vi "Teleop.vi"(10 "Match Info":T1={"Autonomous Elapsed Seconds"=0.0, "TeleOp Elapsed Seconds"=0.0, "Disabled Elapsed Seconds"=0.0, "Visited Autonomous"=FALSE, "Visited TeleOp"=FALSE, "Visited Disabled"=FALSE, "Autonomous Settings"={"Autonomous Style"=enum."Independent", "VI Refnum"=refnum}}, 11 "Call Context":T2) -> ()   [LabVIEW 2016]
doc: "This VI is called for each TeleOp packet received from the DS where the robot is not disabled. It is often used to read from the joysticks and update I/O or to update setpoints for timed control loops. It should complete and return within 20 milliseconds or it may miss DS packets."
uses:
  <vilib>/Rock Robotics/WPI/DriverStation/WPI_DriverStationDerivedRobotMode.ctl
  <vilib>/Rock Robotics/WPI/DriverStation/WPI_DriverStationMatch Info.ctl
  <vilib>/Rock Robotics/WPI/Solenoid/WPI_SolenoidValue.ctl
  <vilib>/Rock Robotics/WPI/Utilities/WPI_GetSetVariantRefNum.vi
  <vilib>/Rock Robotics/Network Tables/NT Write Boolean Array.vi
  <vilib>/Rock Robotics/Network Tables/NT Write Numeric Array.vi
  <vilib>/Rock Robotics/Network Tables/NT Read Boolean.vi
  <vilib>/Rock Robotics/Network Tables/NT Read Number.vi
  <vilib>/Rock Robotics/WPI/Solenoid/WPI_SolenoidSetEnum.vi
  <vilib>/Rock Robotics/Network Tables/NT Write Boolean.vi
  Robot Global Data.vi
  <vilib>/Rock Robotics/WPI/RobotDrive/WPI_RobotDriveArcadeDrive_Standard(NoSaturation).vi
panel:
  out "Sample Slider 0":dbl(slide) scale=0.0..5.0
  out "Sample Boolean 1":bool
  out "Sample Boolean 0":bool
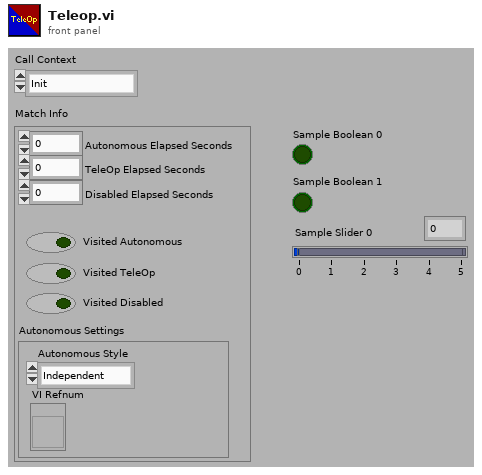
[diagram p1: front panel]
types:
  T1 = typedef "WPI_DriverStationMatch Info.ctl" = cluster{"Autonomous Elapsed Seconds":dbl, "TeleOp Elapsed Seconds":dbl, "Disabled Elapsed Seconds":dbl, "Visited Autonomous":bool, "Visited TeleOp":bool, "Visited Disabled":bool, "Autonomous Settings":cluster{"Autonomous Style":enum16{"Iterative", "Independent"}, "VI Refnum":refnum<vi>}}
  T2 = typedef "WPI_DriverStationDerivedRobotMode.ctl" = enum16{"Init", "Execute", "Stop"}
  T3 = typedef "WPI_SolenoidValue.ctl" = enum16{"Off", "On", "Forward", "Reverse"}
  T4 = typedef "WPI_MotorControlDeviceRef.ctl" = cluster{"DeviceStatus":errorcluster, "Type":T5, "PWM":cluster{"PWM Channel":T6, "DeadBand":T7}, "CAN":cluster{"Device Number":u8, "SetOutput VI Ref":variant, "GetOutput VI Ref":variant, "Enable VI Ref":variant, "Disable VI Ref":variant, "Data":variant}, "Invert":bool}
  T5 = typedef "WPI_MotorControlType.ctl" = enum16{"PWM", "CAN"}
  T6 = typedef "FPGA_DIOPWMChannel.ctl" = enum8{"PWM 0", "PWM 1", "PWM 2", "PWM 3", "PWM 4", "PWM 5", "PWM 6", "PWM 7", "PWM 8", "PWM 9", "PWM MXP 0", "PWM MXP 1", "PWM MXP 2", "PWM MXP 3", "PWM MXP 4", "PWM MXP 5", "PWM MXP 6", "PWM MXP 7", "PWM MXP 8", "PWM MXP 9", "Invalid"}
  T7 = typedef "WPI_PWMDeadband.ctl" = cluster{"Name":string, "maxPositivePwm":i32, "minPositivePwm":i32, "centerPwm":i32, "maxNegativePwm":i32, "minNegativePwm":i32, "angularRange":u16}
  T8 = typedef "WPI_JoystickDevRef.ctl" = cluster{"Device":T9}
  T9 = typedef "WPI_JoystickDeviceEnum.ctl" = enum16{"USB 0", "USB 1", "USB 2", "USB 3", "USB 4", "USB 5"}
  T10 = typedef "WPI_RobotDriveDevRef.ctl" = cluster{"DevStatus":errorcluster, "Motors[]":T4[], "Square Inputs":bool, "Max Output":dbl}
  T11 = typedef "WPI_SolenoidDevRef.ctl" = cluster{"DevStatus":errorcluster, "Pneumatics Control Module":u8, "Forward Solenoid Channel":T12, "Reverse Solenoid Channel":T12}
  T12 = typedef "WPI_SolenoidChannel.ctl" = enum8{"Solenoid 0", "Solenoid 1", "Solenoid 2", "Solenoid 3", "Solenoid 4", "Solenoid 5", "Solenoid 6", "Solenoid 7", "Invalid"}
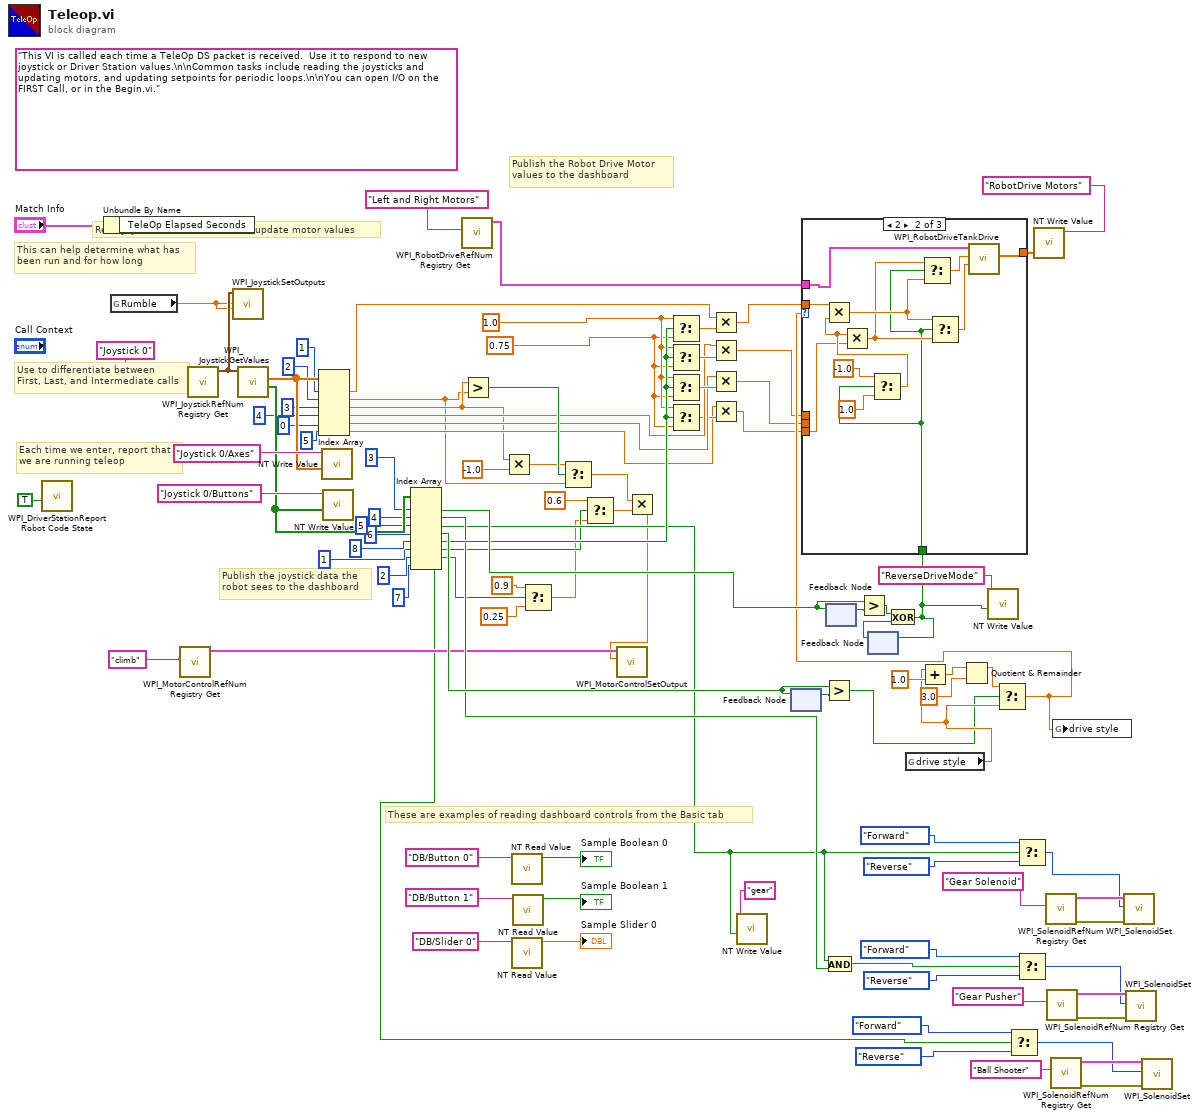
[diagram p0: block diagram]
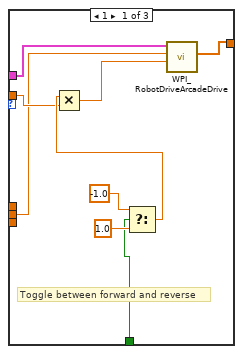
[diagram p2: hidden frame]
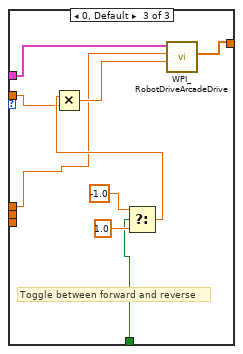
[diagram p3: hidden frame]
diagram:
  w40 = 0.75 ("f")
  w41 = 1.0 ("t")
  (unwired) "This VI is called each time a TeleOp DS packet is received.  Use it to respond to new joystick or Driver Station values.\n\nCommon tasks include reading the joysticks and updating motors, and updating setpoints for periodic loops.\n\nYou can open I/O on the FIRST Call, or in the Begin.vi."
  # "Publish the Robot Drive Motor\nvalues to the dashboard"
  # "These are examples of reading dashboard controls from the Basic tab"
  # "Publish the joystick data the\nrobot sees to the dashboard"
  # "Each time we enter, report that\nwe are running teleop"
  # "Use to differentiate between\nFirst, Last, and Intermediate calls"
  # "This can help determine what has\nbeen run and for how long"
  # "Read Joystick X and Y values and update motor values"
  n1 = call <vilib>:"WPI_DriverStationReport Robot Code State.vi"("TeleOp"=TRUE ("Autonomous")) -> ()  [unwired: 10 in, 1 out]
  n2 = Unbundle By Name("Match Info") -> ()  [unwired: 1 out]
  n3 = global read "Robot Global Data.vi" "Rumble"() -> (w22:dbl)
  n4 = call <vilib>:"WPI_MotorControlRefNum Registry Get.vi"("refnum name"="climb") -> ("MotorControlDevRef"=w16:T4)  [unwired: 9 in, 1 out]
  n5 = call <vilib>:"WPI_JoystickRefNum Registry Get.vi"("refnum name"="Joystick 0") -> ("JoystickDevRef"=w23:T8)  [unwired: 1 in, 9 out]
  n6 = call <vilib>:"WPI_JoystickSetOutputs.vi"("Right Rumble"=w22, "Left Rumble"=w22, "JoystickDevRef"=w23) -> ()  [unwired: 7 in, 2 out]
  n7 = call <vilib>:"WPI_JoystickGetValues.vi"("JoystickDevRef"=w23) -> ("Buttons"=w80:bool[], "Axes"=w96:dbl[])  [unwired: 6 in, 3 out]
  n8 = Index Array(array=w96, index #1=1 ("index"), index #2=2 ("index"), index #3=3 ("index"), index #4=4 ("index"), index #5=0 ("index"), index #6=5 ("index")) -> (element #1=w44:dbl, element #2=w24:dbl, element #3=w25:dbl, element #4=w39:dbl, element #5=w38:dbl, element #6=w36:dbl)
  n9 = call-poly <vilib>:"NT Write Value.vi"("Numeric Array"=w96, "Name"="Joystick 0/Axes") -> ()  [unwired: 9 in, 1 out]
  n10 = call-poly <vilib>:"NT Write Value.vi"("Boolean Array"=w80, "Name"="Joystick 0/Buttons") -> ()  [unwired: 9 in, 1 out]
  n11 = Index Array(array=w80, index #1=3 ("index"), index #2=4 ("index"), index #3=5 ("index"), index #4=6 ("index"), index #5=8 ("index"), index #6=1 ("index"), index #7=2 ("index"), index #8=7 ("index")) -> (element #1=w59:bool, element #2=w28:bool, element #3=w27:bool, element #4=w58:bool, element #5=w45:bool, element #6=w18:bool, element #7=w12:bool, element #8=w1:bool)
  n12 = call <vilib>:"WPI_RobotDriveRefNum Registry Get.vi"("refnum name"="Left and Right Motors") -> ("RobotDriveDevRef"=w75:T10)  [unwired: 1 in, 9 out]
  n13 = Greater?(x=w25, y=w24) -> (0:w62:bool)
  n14 = Multiply(x=w25, y=-1.0) -> (x*y=w26:dbl)
  n15 = call-poly <vilib>:"NT Read Value.vi"("Name"="DB/Button 0" ("refnum name")) -> ("Boolean"=→"Sample Boolean 0":bool)  [unwired: 9 in, 1 out]
  n16 = call-poly <vilib>:"NT Read Value.vi"("Name"="DB/Slider 0" ("refnum name")) -> ("Numeric"=→"Sample Slider 0":dbl)  [unwired: 9 in, 1 out]
  n17 = call-poly <vilib>:"NT Read Value.vi"("Name"="DB/Button 1" ("refnum name")) -> ("Boolean"=→"Sample Boolean 1":bool)  [unwired: 9 in, 1 out]
  n18 = Select(t=0.9, s=w12, f=0.25) -> (s? t:f=w9:dbl)
  n19 = Select(t=w26, s=w62, f=w24) -> (s? t:f=w20:dbl)
  n20 = Select(t=0.6, s=w18, f=w9) -> (s? t:f=w21:dbl)
  n21 = Multiply(x=w20, y=w21) -> (x*y=w13:dbl)
  n22 = call <vilib>:"WPI_MotorControlSetOutput.vi"("Output"=w13, "MotorControlDevRef"=w16) -> ()  [unwired: 7 in, 3 out]
  n23 = Select(t=w41, s=w45, f=w40) -> (s? t:f=w47:dbl)
  n24 = Select(t=w41, s=w45, f=w40) -> (s? t:f=w43:dbl)
  n25 = Select(t=w41, s=w45, f=w40) -> (s? t:f=w42:dbl)
  n26 = Select(t=w41, s=w45, f=w40) -> (s? t:f=w37:dbl)
  n27 = Multiply(x=w44, y=w47) -> (x*y=w46:dbl)
  n28 = Multiply(x=w39, y=w43) -> (x*y=w35:dbl)
  n29 = Multiply(x=w38, y=w42) -> (x*y=w34:dbl)
  n30 = Multiply(x=w36, y=w37) -> (x*y=w33:dbl)
  n31 = call-poly <vilib>:"NT Write Value.vi"("Boolean"=w27, "Name"="gear") -> ()  [unwired: 9 in, 1 out]
  n32 = feedback #1() -> (w60:bool)  [unwired: 1 in]
  n33 = feedback-in #1(w58) -> ()
  n34 = Greater?(x=w58, y=w60) -> (0:w50:bool)
  n35 = And(x=w27, y=w28) -> (x .and. y?=w29:bool)
  n36 = feedback #2() -> (w69:bool)  [unwired: 1 in]
  n37 = feedback-in #2(w59) -> ()
  n38 = Greater?(x=w59, y=w69) -> (0:w68:bool)
  n39 = feedback #3() -> (w70:bool)  [unwired: 1 in]
  n40 = Exclusive Or(1:w70, 2:w68) -> (0:w67:bool)
  n41 = feedback-in #3(w67) -> ()
  n42 = global read "Robot Global Data.vi" "drive style"() -> (w56:dbl)
  n43 = Add(x=w56, y=1.0) -> (x+y=w53:dbl)
  n44 = Quotient & Remainder(x=w53, y=3.0) -> (x-y*floor(x/y)=w55:dbl)  [unwired: 1 out]
  n45 = call-poly <vilib>:"NT Write Value.vi"("Boolean"=w67, "Name"="ReverseDriveMode") -> ()  [unwired: 9 in, 1 out]
  n46 = Select(t=w55, s=w50, f=w56) -> (s? t:f=w52:dbl)
  n47 = case shown="2" w52 {
    tunnel: w75 -> [w110 w115 w131]
    tunnel: w46 -> [w104 w114 w124]
    tunnel: [w111 w112 w132] -> w73
    tunnel: w35 -> [_ _ w125]
    tunnel: w67 -> [w105 w116 w126]
    tunnel: w34 -> [w103 _ _]
    tunnel: w33 -> [_ w113 _]
    frame 1 {
      # "Toggle between forward and reverse"
      n48 = Select(t=-1.0, s=w105, f=1.0) -> (s? t:f=w107:dbl)
      n49 = Multiply(x=w107, y=w104) -> (x*y=w106:dbl)
      n50 = call-poly <vilib>:"WPI_RobotDriveArcadeDrive.vi"("Y axis value"=w106, "X axis value"=w103, "RobotDriveDevRef"=w110) -> ("Motor Values"=w111:dbl[])  [unwired: 6 in, 2 out]
    }
    frame 2 {
      n51 = Select(t=-1.0, s=w116, f=1.0) -> (s? t:f=w117:dbl)
      n52 = Multiply(x=w114, y=w117) -> (x*y=w120:dbl)
      n53 = Multiply(x=w117, y=w113) -> (x*y=w118:dbl)
      n54 = Select(t=w118, s=w116, f=w120) -> (s? t:f=w119:dbl)
      n55 = Select(t=w120, s=w116, f=w118) -> (s? t:f=w121:dbl)
      n56 = call <vilib>:"WPI_RobotDriveTankDrive.vi"("Right axis value"=w121, "Left axis value"=w119, "RobotDriveDevRef"=w115) -> ("Motor Values"=w112:dbl[])  [unwired: 6 in, 2 out]
    }
    frame 0, Default {
      # "Toggle between forward and reverse"
      n57 = Select(t=-1.0, s=w126, f=1.0) -> (s? t:f=w128:dbl)
      n58 = Multiply(x=w128, y=w124) -> (x*y=w127:dbl)
      n59 = call-poly <vilib>:"WPI_RobotDriveArcadeDrive.vi"("Y axis value"=w127, "X axis value"=w125, "RobotDriveDevRef"=w131) -> ("Motor Values"=w132:dbl[])  [unwired: 6 in, 2 out]
    }
  }
  n60 = Select(t=WPI_SolenoidValue."Forward" ("Value"), s=w1, f=WPI_SolenoidValue."Reverse" ("Value")) -> (s? t:f=w2:T3)
  n61 = Select(t=WPI_SolenoidValue."Forward" ("Value"), s=w27, f=WPI_SolenoidValue."Reverse" ("Value")) -> (s? t:f=w82:T3)
  n62 = Select(t=WPI_SolenoidValue."Forward" ("Value"), s=w29, f=WPI_SolenoidValue."Reverse" ("Value")) -> (s? t:f=w30:T3)
  n63 = call-poly <vilib>:"NT Write Value.vi"("Numeric Array"=w73, "Name"="RobotDrive Motors") -> ()  [unwired: 9 in, 1 out]
  n64 = call <vilib>:"WPI_SolenoidRefNum Registry Get.vi"("refnum name"="Gear Solenoid") -> ("error out"=w89:errorcluster, "SolenoidDevRef"=w90:T11)  [unwired: 9 in]
  n65 = call <vilib>:"WPI_SolenoidRefNum Registry Get.vi"("refnum name"="Gear Pusher") -> ("error out"=w84:errorcluster, "SolenoidDevRef"=w85:T11)  [unwired: 9 in]
  n66 = call <vilib>:"WPI_SolenoidRefNum Registry Get.vi"("refnum name"="Ball Shooter") -> ("error out"=w5:errorcluster, "SolenoidDevRef"=w6:T11)  [unwired: 9 in]
  n67 = global write "Robot Global Data.vi" "drive style"(w52) -> ()
  n68 = call-poly <vilib>:"WPI_SolenoidSet.vi"("error in (no error)"=w89, "Value"=w82, "SolenoidDevRef"=w90) -> ()  [unwired: 7 in, 2 out]
  n69 = call-poly <vilib>:"WPI_SolenoidSet.vi"("error in (no error)"=w84, "Value"=w30, "SolenoidDevRef"=w85) -> ()  [unwired: 7 in, 2 out]
  n70 = call-poly <vilib>:"WPI_SolenoidSet.vi"("error in (no error)"=w5, "Value"=w2, "SolenoidDevRef"=w6) -> ()  [unwired: 7 in, 2 out]
